vi "Get Size of Data from TD - Cluster of Error Clusters - Returns Correct Size.vi"() -> ()   [LabVIEW 2017, in "Composition.Tests.lvlib"]
uses:
  Composition.Tests.lvlib
  <vilib>/addons/_JKI Toolkits/Caraya/classes/Assert/Assert Equal Value_Variant.vi
  Composition/Composition.lvlib
  <vilib>/addons/_JKI Toolkits/Caraya/classes/Assert/Assert.lvclass
  <vilib>/addons/_JKI Toolkits/Caraya/classes/Test/Test.lvclass
panel:
  out "error out":errorcluster
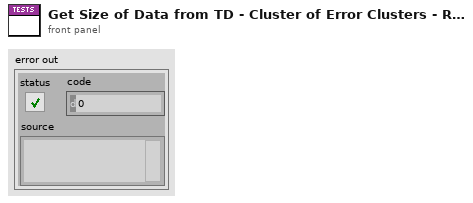
[diagram p1: front panel]
types:
  T1 = cluster{"error constant":errorcluster, "error constant 2":errorcluster, "error constant 3":errorcluster}
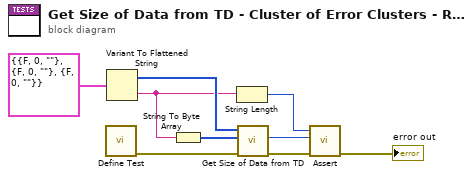
[diagram p0: block diagram]
diagram:
  n1 = call <vilib>:"Define Test.vi"() -> ("error out"=w2:errorcluster)  [unwired: 11 in]
  n2 = Variant To Flattened String(Variant=T1 {"error constant"={"status"=FALSE, "code"=0, "source"=""}, "error constant 2"={"status"=FALSE, "code"=0, "source"=""}, "error constant 3"={"status"=FALSE, "code"=0, "source"=""}}) -> (data string=w6:string, 1:w9:i16[])
  n3 = String To Byte Array(string=w6) -> (unsigned byte array=w8:u8[])
  n4 = String Length(string=w6) -> (length=w3:i32)
  n5 = call "Get Size of Data from TD.vi"("error in (no error)"=w2, "Data String"=w8, "Type Descriptor"=w9) -> ("error out"=w7:errorcluster, "Size of Data"=w4:i32)  [unwired: 7 in]
  n6 = call-poly <vilib>:"Assert.vi"("error in (no error)"=w7, "Y"=w4, "X"=w3) -> ("error out"=→"error out":errorcluster)  [unwired: 8 in]
